vi "Generate PXITrigger.vi"(6 "duration (ticks)":u32=25, 7 "Trigger IO":refnum<k21>, 8 "enable trigger generation":bool, 11 "send trigger":bool) -> (3 "generated trig":bool)   [LabVIEW 2019, in "FPGA Utility.lvlib"]
doc: "Generate PXI trigger with defined duration (in clock ticks) on specified line"
uses:
  FPGA Utility.lvlib
  <vilib>/rvi/eio/common/nirviEmuTemplateMethod_errors.vi
  <vilib>/eio/EIOMethodNode/EIOMethodNode.xnode
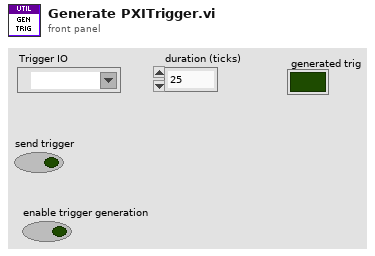
[diagram p1: front panel]
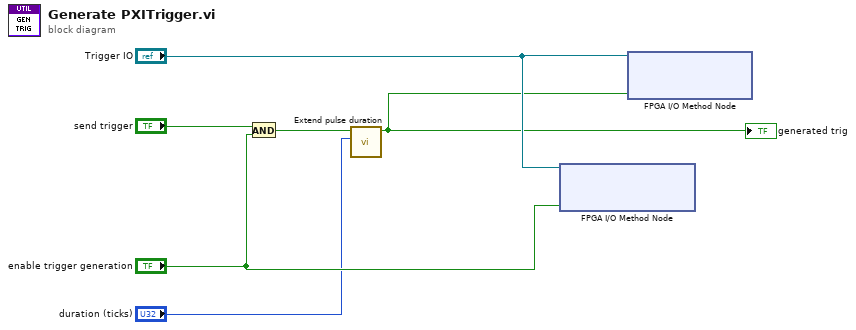
[diagram p0: block diagram]
diagram:
  n1 = And(x="send trigger", y="enable trigger generation") -> (x .and. y?=w4:bool)
  n2 = call "Extend pulse duration.vi"("duration (ticks)"="duration (ticks)", "Boolean"=w4) -> ("out"=w1:bool)  [unwired: 9 in]
  "generated trig" <- w1
  n3 = xnode "FPGA I/O Method Node"("FPGA I/O In"="Trigger IO", "Enable"="enable trigger generation") -> ()  [unwired: 1 out]
  n4 = xnode "FPGA I/O Method Node"("FPGA I/O In"="Trigger IO", "Data"=w1) -> ()  [unwired: 1 out]
